vi "FPGA_WriteAO.vi"(8 "error in":errorcluster, 10 "Voltage":dbl min=0.0 max=5.0, 11 "AO Reference":T1={"DevStatus"={"status"=FALSE, "code"=0, "source"=""}, "AO Channel"=enum."Invalid"}) -> (0 "error out":errorcluster, 3 "AO Reference":T1={"DevStatus"={"status"=FALSE, "code"=0, "source"=""}, "AO Channel"=enum."Invalid"})   [LabVIEW 2017]
uses:
  <vilib>/Rock Robotics/WPI/AnalogOutput/WPI_AOChannelDevRef.ctl
  <vilib>/Rock Robotics/WPI/AnalogOutput/WPI_AnalogOutputChannel.ctl
  <vilib>/Rock Robotics/SystemInterfaces/System/FPGA_SystemFPGA Ref Global.vi
  <vilib>/Utility/error.llb/Error Cluster From Error Code.vi
  <vilib>/rvi/errors/niLvFpgaAdjustHostInterfaceError.vi
  <vilib>/rvi/interface/nirviReadWriteControl/nirviReadWriteControl.xnode
  <vilib>/Rock Robotics/SystemInterfaces/System/FPGA_SystemFRC FPGA Ref.ctl
  NiFpgaLv.dll
  <vilib>/rvi/interface/Simulation/niFpgaSimulationCallBeginRW.vi
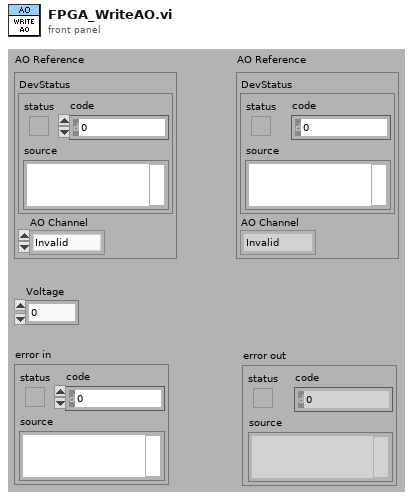
[diagram p1: front panel]
types:
  T1 = typedef "WPI_AOChannelDevRef.ctl" = cluster{"DevStatus":errorcluster, "AO Channel":T2}
  T2 = typedef "WPI_AnalogOutputChannel.ctl" = enum8{"AO MXP 0", "AO MXP 1", "Invalid"}
  T3 = typedef "FPGA_SystemFRC FPGA Ref.ctl" = refnum<k20>
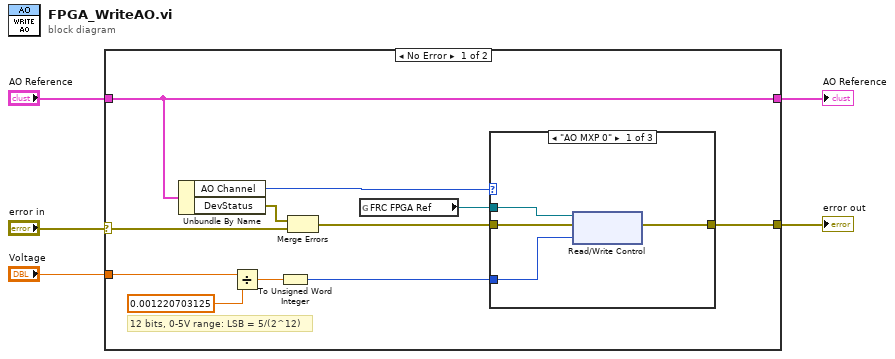
[diagram p0: block diagram]
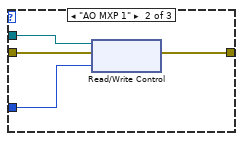
[diagram p2: hidden frame]
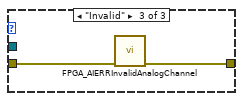
[diagram p3: hidden frame]
diagram:
  n1 = case shown="No Error" "error in" {
    selector: "error in" -> [w7 w27]
    tunnel: [w16 w27] -> w5
    tunnel: "AO Reference" -> [w8 w28]
    tunnel: "Voltage" -> [w12 _]
    tunnel: [w8 w28] -> w1
    frame No Error {
      # "12 bits, 0-5V range: LSB = 5/(2^12)"
      n2 = Unbundle By Name(w8) -> ("AO Channel"=w13:T2, "DevStatus"=w14:errorcluster)
      n3 = Divide(x=w12, y=0.001220703125 ("12 bits, 0-5V range: LSB = 5/(2^12)")) -> (x/y=w10:dbl)
      n4 = To Unsigned Word Integer(number=w10) -> (unsigned 16bit integer=w9:u16)
      n5 = Merge Errors(w14, w7) -> (w15:errorcluster)
      n6 = global read "FPGA_SystemFPGA Ref Global.vi" "FRC FPGA Ref"() -> (w6:T3)
      n7 = case shown="\"AO MXP 0\"" w13 {
        tunnel: w6 -> [w18 w22 _]
        tunnel: w15 -> [w20 w24 w26]
        tunnel: [w19 w23 w25] -> w16
        tunnel: w9 -> [w17 w21 _]
        frame "AO MXP 0" {
          n8 = xnode "Read/Write Control"("FPGA VI Reference In"=w18, "error in"=w20, "AO.MXP0"=w17) -> ("error out"=w19:errorcluster)  [unwired: 1 out]
        }
        frame "AO MXP 1" {
          n9 = xnode "Read/Write Control"("FPGA VI Reference In"=w22, "error in"=w24, "AO.MXP1"=w21) -> ("error out"=w23:errorcluster)  [unwired: 1 out]
        }
        frame "Invalid" {
          n10 = call <vilib>:"FPGA_AIERRInvalidAnalogChannel.vi"("error in (no error)"=w26) -> ("error out"=w25:errorcluster)  [unwired: 10 in]
        }
      }
    }
    frame Error {
    }
  }
  "AO Reference" <- w1
  "error out" <- w5
